vi "Handle Errors.vi"(8 "error in":errorcluster, 11 "CRDS in":refnum<class "CRDS.lvclass">=refnum) -> (0 "error out":errorcluster, 2 "errors":errorcluster[](array[cluster]), 3 "CRDS out":refnum<class "CRDS.lvclass">)   [LabVIEW 2014, in "CRDS.lvclass"]
uses:
  CRDS.lvclass
  Instrument/Instrument.lvclass
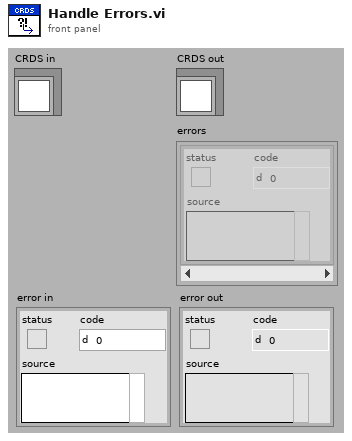
[diagram p1: front panel]
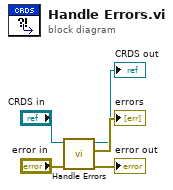
[diagram p0: block diagram]
diagram:
  n1 = call-parent "Handle Errors.vi"("error in"="error in", "Instrument in"="CRDS in") -> ("error out"=→"error out":errorcluster, "errors"=→"errors":errorcluster[], "Instrument out"=→"CRDS out":refnum<class "Instrument.lvclass">)  [unwired: 7 in]
